vi "Przenies nazwy wykresow FVG.vi"(7 "Akcja (GET)":T1, 8 "error in (no error)":errorcluster, 9 "Wykres 3 in":string[](array[string]), 10 "Wykres 2 in":string[](array[string]), 11 "Wykres 1 in":string[](array[string])) -> (0 "error out":errorcluster, 1 "Wykres 3 out":string[](array[string]), 2 "Wykres 2 out":string[](array[string]), 3 "Wykres 1 out":string[](array[string]), 4 "Zmieniono?":bool)   [LabVIEW 2014]
doc: "Przenosi nazwy wybranych 2 wykresów\ndo pêtli wyœwietlania"
uses:
  Kontrolki/FVGs/FVG akcje podstawowa.ctl
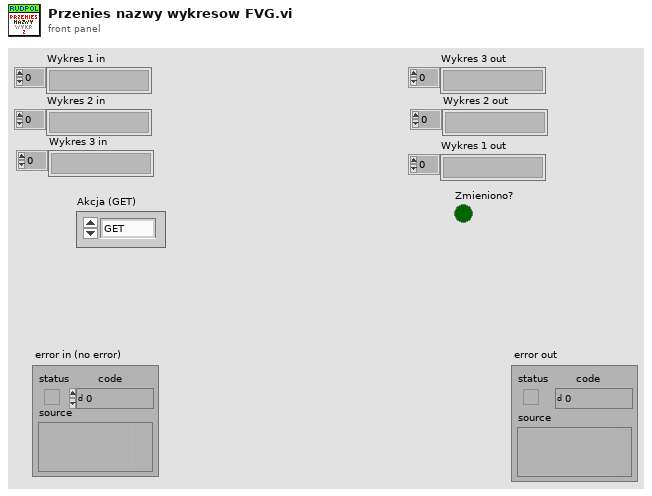
[diagram p1: front panel]
types:
  T1 = typedef "FVG akcje podstawowa.ctl" = enum16{"GET", "SET"}
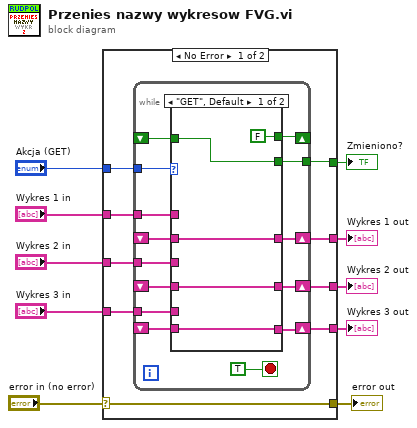
[diagram p0: block diagram]
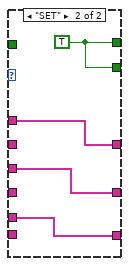
[diagram p2: hidden frame]
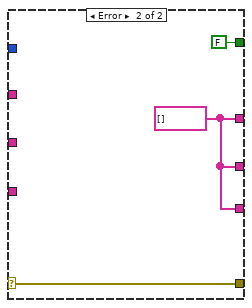
[diagram p3: hidden frame]
diagram:
  n1 = case shown="No Error" "error in (no error)" {
    selector: "error in (no error)" -> [w15 w45]
    tunnel: [w15 w45] -> w9
    tunnel: "Wykres 1 in" -> [w19 _]
    tunnel: "Wykres 2 in" -> [w18 _]
    tunnel: "Wykres 3 in" -> [w17 _]
    tunnel: "Akcja (GET)" -> [w16 _]
    tunnel: [w14 w44] -> w4
    tunnel: [w13 w44] -> w3
    tunnel: [w12 w44] -> w2
    tunnel: [w11 FALSE] -> w1
    frame No Error {
      n2 = while {
        tunnel: w19 -> [w31]
        tunnel: w18 -> [w30]
        tunnel: w17 -> [w29]
        tunnel: w16 -> [w32]
        shift-right: [w28] -> w12
        shift-left: _ -> [w27]
        shift-right: [w26] -> w13
        shift-left: _ -> [w25]
        shift-right: [w24] -> w14
        shift-left: _ -> [w23]
        shift-right: [w22] -> _
        shift-left: _ -> [w20]
        tunnel: [w21] -> w11
        stop <- TRUE stop-if-true
        n3 = case shown="\"GET\", Default" w32 {
          tunnel: w31 -> [_ w42]
          tunnel: w30 -> [_ w41]
          tunnel: w29 -> [_ w40]
          tunnel: [w38 w42] -> w28
          tunnel: w27 -> [w38 _]
          tunnel: [w37 w41] -> w26
          tunnel: w25 -> [w37 _]
          tunnel: [w36 w40] -> w24
          tunnel: w23 -> [w36 _]
          tunnel: [FALSE w39] -> w22
          tunnel: [w35 w39] -> w21
          tunnel: w20 -> [w35 _]
          frame "GET", Default {
          }
          frame "SET" {
            w39 = TRUE
          }
        }
      }
    }
    frame Error {
      w44 = string[] [] ("Wykres 1 in")
    }
  }
  "error out" <- w9
  "Wykres 3 out" <- w4
  "Wykres 2 out" <- w3
  "Wykres 1 out" <- w2
  "Zmieniono?" <- w1
